vi "selections.load.binaries.vi"(8 "error in (no error)":errorcluster, 10 "filters":T1, 11 "manager_daemon":refnum<class "manager_daemon.lvclass">) -> (0 "error out":errorcluster, 2 "filters out":T1, 3 "manager_daemon out":refnum<class "manager_daemon.lvclass">)   [LabVIEW 2024]
uses:
  comic_manager/manager_daemon/manager_daemon.lvclass
  selection_dropdown/selection_dropdown.lvclass
  comic_manager/manager_daemon/type_defs/sub-map--map.ctl
  comic_manager/manager_daemon/type_defs/SubData--cluster.ctl
  comic_manager/manager_daemon/manager_daemon.lvclass/manager_daemon.ctl
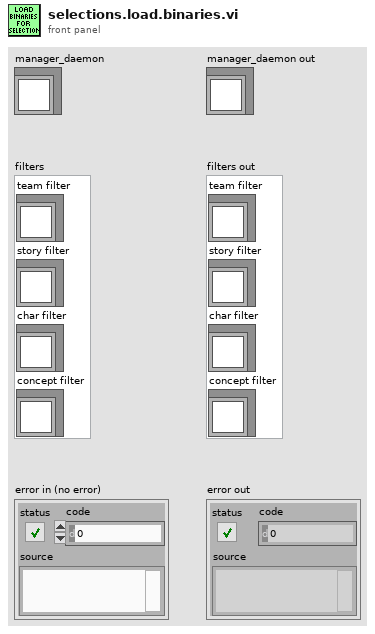
[diagram p1: front panel]
types:
  T1 = cluster{"team filter":refnum<class "selection_dropdown.lvclass">, "story filter":refnum<class "selection_dropdown.lvclass">, "char filter":refnum<class "selection_dropdown.lvclass">, "concept filter":refnum<class "selection_dropdown.lvclass">}
  T2 = typedef "manager_daemon.lvclass/sub-map--map.ctl" = map{string, T3}
  T3 = typedef "manager_daemon.lvclass/SubData--cluster.ctl" = cluster{"id":i32, "issues":set{i32}}
  T4 = typedef "manager_daemon.lvclass/paths--cluster.ctl" = cluster{"issue map path":path, "char map path":path, "concept map path":path, "story map path":path, "team map path":path, "volume map path":path, "volumes path":path, "issues path":path}
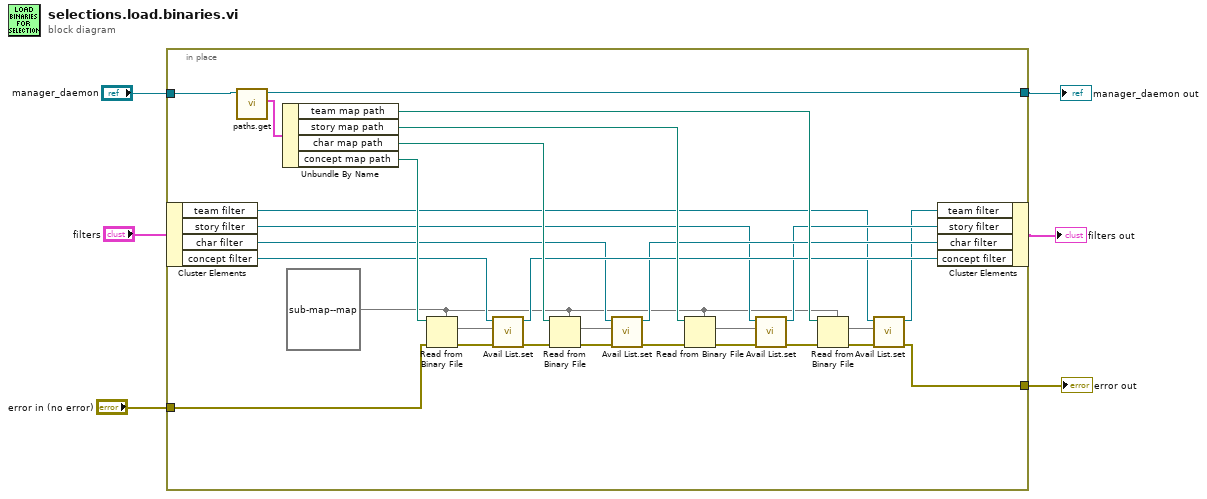
[diagram p0: block diagram]
diagram:
  n1 = in-place {
    in-place-border: "error in (no error)" -> [w10]
    in-place-border: [w9] -> w5
    in-place-border: "manager_daemon" -> [w8]
    in-place-border: [w7] -> w3
    w11 = T2 {} ("char map")
    n2 = in-place-cluster #1("filters") -> ("team filter"=w16:refnum<class "selection_dropdown.lvclass">, "story filter"=w19:refnum<class "selection_dropdown.lvclass">, "char filter"=w21:refnum<class "selection_dropdown.lvclass">, "concept filter"=w27:refnum<class "selection_dropdown.lvclass">)
    n3 = call "paths.get.vi"("manager_daemon in"=w8) -> ("paths"=w35:T4, "manager_daemon out"=w7:refnum<class "manager_daemon.lvclass">)  [unwired: 9 in]
    n4 = Unbundle By Name(w35) -> ("team map path"=w34:path, "story map path"=w31:path, "char map path"=w32:path, "concept map path"=w33:path)
    n5 = Read from Binary File(5:w11, 8:w10, 11:w33) -> (0:w30:errorcluster, 2:w28:T2)  [unwired: 3 in, 2 out]
    n6 = call-dynamic "Avail List.set.vi"("error in (no error)"=w30, "detail map"=w28, "selection_dropdown in"=w27) -> ("error out"=w29:errorcluster, "selection_dropdown out"=w26:refnum<class "selection_dropdown.lvclass">)  [unwired: 7 in]
    n7 = Read from Binary File(5:w11, 8:w29, 11:w32) -> (0:w25:errorcluster, 2:w12:T2)  [unwired: 3 in, 2 out]
    n8 = call-dynamic "Avail List.set.vi"("error in (no error)"=w25, "detail map"=w12, "selection_dropdown in"=w21) -> ("error out"=w24:errorcluster, "selection_dropdown out"=w20:refnum<class "selection_dropdown.lvclass">)  [unwired: 7 in]
    n9 = Read from Binary File(5:w11, 8:w24, 11:w31) -> (0:w23:errorcluster, 2:w13:T2)  [unwired: 3 in, 2 out]
    n10 = call-dynamic "Avail List.set.vi"("error in (no error)"=w23, "detail map"=w13, "selection_dropdown in"=w19) -> ("error out"=w22:errorcluster, "selection_dropdown out"=w18:refnum<class "selection_dropdown.lvclass">)  [unwired: 7 in]
    n11 = Read from Binary File(5:w11, 8:w22, 11:w34) -> (0:w17:errorcluster, 2:w14:T2)  [unwired: 3 in, 2 out]
    n12 = call-dynamic "Avail List.set.vi"("error in (no error)"=w17, "detail map"=w14, "selection_dropdown in"=w16) -> ("error out"=w9:errorcluster, "selection_dropdown out"=w15:refnum<class "selection_dropdown.lvclass">)  [unwired: 7 in]
    n13 = in-place-cluster #1("team filter"=w15, "story filter"=w18, "char filter"=w20, "concept filter"=w26) -> (→"filters out":T1)
  }
  "error out" <- w5
  "manager_daemon out" <- w3
